vi "userauth_authenticated.vi"() -> ()   [LabVIEW 2013]
doc: "Illustrates how to verify that the current session is authenticated."
uses:
  libssh2/libssh2_init_default.vi
  libssh2/libssh2_session_handshake_tcp.vi
  libssh2/libssh2.lvlib
panel:
  out "authenticated (after login)":bool
  out "authenticated (before login)":bool
  in  "password":string
  in  "username":string
  in  "hostname":string="localhost"
  out "error out":errorcluster
  # "Note: this value should be FALSE as\nwe are not authenticated."
  # "Note: this value should be TRUE as\nwe are authenticated."
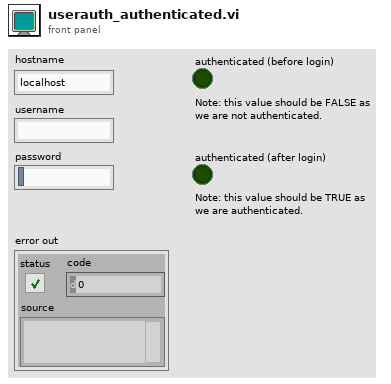
[diagram p1: front panel]
types:
  T1 = typedef "libssh2.lvlib/Session Refnum.ctl" = refnum<k1>
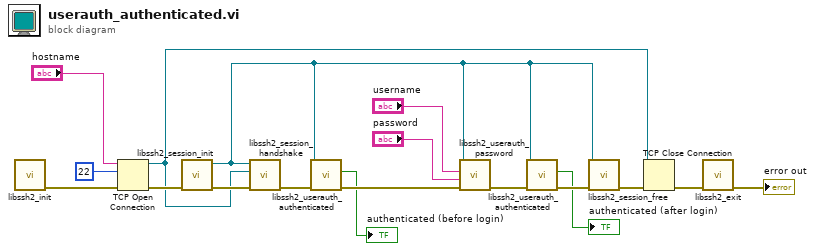
[diagram p0: block diagram]
diagram:
  n1 = call-poly "libssh2_init.vi"() -> ("error out"=w18:errorcluster)  [unwired: 11 in]
  n2 = TCP Open Connection(address="hostname", remote port or service name=u16 22, error in (no error)=w18) -> (connection ID=w7:refnum<k5>, error out=w8:errorcluster)  [unwired: 2 in]
  n3 = call "libssh2_session_init.vi"("error in (no error)"=w8) -> ("error out"=w13:errorcluster, "session"=w3:T1)  [unwired: 9 in]
  n4 = call-poly "libssh2_session_handshake.vi"("error in (no error)"=w13, "tcp connection"=w7, "session"=w3) -> ("error out"=w12:errorcluster)  [unwired: 8 in]
  n5 = call "libssh2_userauth_authenticated.vi"("error in (no error)"=w12, "session"=w3) -> ("error out"=w5:errorcluster, "authenticated"=→"authenticated (before login)":bool)  [unwired: 8 in]
  n6 = call "libssh2_userauth_password.vi"("error in (no error)"=w5, "password"="password", "username"="username", "session"=w3) -> ("error out"=w6:errorcluster)  [unwired: 7 in]
  n7 = call "libssh2_userauth_authenticated.vi"("error in (no error)"=w6, "session"=w3) -> ("error out"=w4:errorcluster, "authenticated"=→"authenticated (after login)":bool)  [unwired: 8 in]
  n8 = call "libssh2_session_free.vi"("error in (no error)"=w4, "session"=w3) -> ("error out"=w9:errorcluster)  [unwired: 9 in]
  n9 = TCP Close Connection(connection ID=w7, error in (no error)=w9) -> (error out=w15:errorcluster)  [unwired: 1 in, 1 out]
  n10 = call "libssh2_exit.vi"("error in (no error)"=w15) -> ("error out"=→"error out":errorcluster)  [unwired: 10 in]
